vi "FFT Spectrum (Real-Im) for N Chan.vi"(4 "window parameter":dbl=nan, 6 "averaging parameters":T3={"averaging mode"=enum."No averaging", "weighting mode"=enum."Exponential", "number of averages"=10} {"number of averages" min=1}, 7 "restart averaging (F)":bool, 8 "error in (no error)":errorcluster, 10 "window":T2=1 items=["Rectangle"=0, "Hanning"=1, "Hamming"=2, "Blackman-Harris"=3, "Exact Blackman"=4, "Blackman"=5, "Flat Top"=6, "4 Term B-Harris "=7, "7 Term B-Harris"=8, "Low Sidelobe"=9, "Blackman Nuttall"=11, "Triangle"=30, "Bartlett-Hanning"=31, "Bohman"=32, "Parzen"=33, "Welch"=34, "Kaiser"=60, "Dolph-Chebyshev"=61, "Gaussian"=62], 11 "time signals":waveform(dbl)[](array[waveform])) -> (0 "error out":errorcluster, 1 "averages completed":dbl, 2 "imaginary parts":T1(array[cluster]) {"imaginary part" format="%0.2f"; "f0" format="%.2p"; "df" format="%.2p"}, 3 "real parts":cluster{"f0":dbl, "df":dbl, "real part":dbl[]}[](array[cluster]) {"real part" format="%.2p"; "f0" format="%.2p"; "df" format="%.2p"}, 5 "averaging done":bool)   [LabVIEW 2020, in "NI_MAPro.lvlib"]
doc: "Computes the averaged FFT spectrum of <B>time signal</B>. This VI returns the FFT results as real and imaginary parts. Wire data to the <B>time signal</B> input to determine the polymorphic instance to use or manually select the instance."
uses:
  NI_MAPro.lvlib
  windowTd.ctl
  NI_MABase.lvlib
  NI_AALPro.lvlib
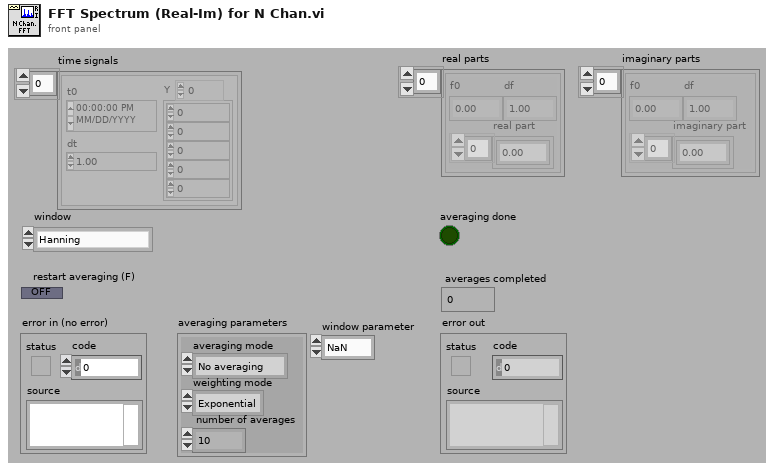
[diagram p1: front panel]
types:
  T1 = cluster{"f0":dbl, "df":dbl, "imaginary part":dbl[]}[]
  T2 = typedef "NI_AALPro.lvlib/windowTd.ctl" = u32
  T3 = cluster{"averaging mode":enum16{"No averaging", "Vector averaging", "RMS averaging", "Peak hold"}, "weighting mode":enum16{"Linear", "Exponential"}, "number of averages":u32}
  T4 = cluster{"block size":i32, "dt":dbl, "spectrum parameters":cluster{"averaging parameters":cluster{"averaging mode":enum16{"No averaging", "Vector averaging", "RMS averaging", "Peak hold"}, "weighting mode":enum16{"Linear", "Exponential"}, "number of averages":u32}, "window":T2}, "df":dbl, "averages completed":dbl, "complex spectrum":cdb[], "real spectrum":dbl[], "t0 history":dbl, "dt history":dbl, "timestamp":dbl, "lin avg done":bool}
  T5 = cluster{"dB On (F)":bool, "unwrap phase (F)":bool, "convert to degree (F)":bool}
  T6 = cluster{"f0":dbl, "df":dbl, "imag or phase":dbl[]}
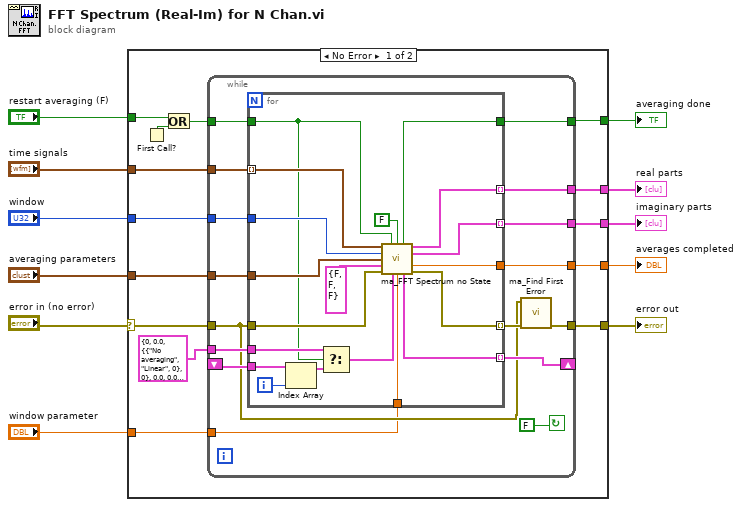
[diagram p0: block diagram]
diagram:
  n1 = case shown="No Error" "error in (no error)" {
    selector: "error in (no error)" -> [w22 w61]
    tunnel: [w24 w61] -> w11
    tunnel: "window parameter" -> [w20 _]
    tunnel: "restart averaging (F)" -> [w19 _]
    tunnel: "time signals" -> [w18 _]
    tunnel: "window" -> [w17 _]
    tunnel: "averaging parameters" -> [w16 _]
    tunnel: [w15 _] -> w4
    tunnel: [w14 _] -> w3
    tunnel: [w13 _] -> w2
    tunnel: [w12 _] -> w1
    frame No Error {
      n2 = First Call?() -> (First Call?: T/F=w25:bool)
      n3 = Or(x=w19, y=w25) -> (x .or. y?=w23:bool)
      n4 = while {
        tunnel: [w41] -> w15
        tunnel: [w40] -> w12
        tunnel: [w39] -> w14
        tunnel: [w28] -> w24
        shift-right: [w37] -> _
        shift-left: _ -> [w36]
        tunnel: w23 -> [w34]
        tunnel: w18 -> [w33]
        tunnel: w17 -> [w32]
        tunnel: w16 -> [w31]
        tunnel: w22 -> [w27]
        tunnel: [w30] -> w13
        tunnel: T4 {"block size"=0, "dt"=0.0, "spectrum parameters"={"averaging parameters"={"averaging mode"=enum."No averaging", "weighting mode"=enum."Linear", "number of averages"=0}, "window"=0}, "df"=0.0, "averages completed"=0.0, "complex spectrum"=[], "real spectrum"=[], "t0 history"=0.0, "dt history"=0.0, "timestamp"=0.0, "lin avg done"=FALSE} ("state info") -> [w29]
        tunnel: w20 -> [w26]
        stop <- FALSE continue-if-true
        n5 = for {
          tunnel: [w60] -> w41
          tunnel: [w59] -> w40
          tunnel: [w58] -> w39 mode=indexing
          tunnel: [w57] -> w38 mode=indexing
          tunnel: [w56] -> w37 mode=indexing
          tunnel: w36 -> [w54]
          tunnel: w34 -> [w44]
          tunnel: w33 -> [w50] mode=indexing
          tunnel: w32 -> [w49]
          tunnel: w31 -> [w48]
          tunnel: w27 -> [w47]
          tunnel: [w46] -> w30 mode=indexing
          tunnel: w29 -> [w45]
          tunnel: w26 -> [w42]
          i -> [w53]
          n6 = Index Array(array=w54, index=w53) -> (element=w52:T4)
          n7 = Select(t=w45, s=w44, f=w52) -> (s? t:f=w55:T4)
          n8 = call "ma_FFT Spectrum no State.vi"("time signal"=w50, "restart averaging (F)"=w44, "mag-phase"=FALSE, "window"=w49, "averaging parameters"=w48, "view"=T5 {"dB On (F)"=FALSE, "unwrap phase (F)"=FALSE, "convert to degree (F)"=FALSE}, "error in"=w47, "state info"=w55, "window parameter"=w42) -> ("averaging done"=w60:bool, "real or mag"=w58:cluster{"f0":dbl, "df":dbl, "real or mag":dbl[]}, "imag or phase"=w46:T6, "averages completed"=w59:dbl, "state info"=w56:T4, "error out"=w57:errorcluster)  [unwired: 1 out]
        }
        n9 = call "ma_Find First Error.vi"("error array in"=w38, "error in 1 (no error)"=w27) -> ("error out"=w28:errorcluster)  [unwired: 2 in, 3 out]
      }
    }
    frame Error {
    }
  }
  "error out" <- w11
  "averages completed" <- w1
  "averaging done" <- w4
  "imaginary parts" <- w2
  "real parts" <- w3
